vi "Combine_Anomaly_Detection_Results.vi"(4 "Relative Resolution":sgl=1.0, 5 "Evaluation_Results":T7={"Threshold(Image)"=-1.0, "Threshold(Pixel)"=-1.0, "Pixel_Range"={"Min"=-1.0, "Max"=-1.0}} {"Pixel_Range"."Min" format="%#_5g"}, 6 "Display_Options":T1={"ROI_Options"={"Color"=16711680, "Width"=3, "Drawing Mode"=enum."Frame"}, "Heatmap_Options"={"ColorMap"=enum."Jet", "Alpha"=0.4, "Heatmap Range"={"Min"=-1.0, "Max"=-1.0}}, "Has GT?"=FALSE} {"Heatmap_Options"."Heatmap Range"."Min" format="%#_5g"}, 7 "Pixel Anomaly Thrshld":sgl=26.0 format="%_4g", 8 "error in":errorcluster, 9 "Anomaly Map":sgl[][](array[numeric]), 10 "Gt File Path":path, 11 "Orig Image In":T6=refnum) -> (0 "error out":errorcluster, 2 "Actual Pixel Threshold":sgl=26.0, 3 "Anomaly Detection Rresults":T8={"Image"="remote image 000002ADCD8F5788", "Ground Truth"=refnum, "Predicted Heat Map"="remote image 000002ADCD8F5838", "Predicted Mask"="remote image 000002ADCD8F5A48", "Segmentation"=refnum})   [LabVIEW 2020]
uses:
  Controls/Anomaly_Detection_Results_Imgs.ctl
  <vilib>/Ngene/DeepLTK Anomaly Detection Addon/DeepLTK_Anomaly_Detection_Addon/API/Controls/NNPC_Evaluation_Results.ctl
  <vilib>/vision/Image Controls.llb/IMAQ Image.ctl
  Controls/Display_Options.ctl
  Controls/ROI_Display_Options.ctl
  Controls/Heatmap_Display_Options.ctl
  Controls/ColorMap.ctl
  <vilib>/Ngene/DeepLTK Anomaly Detection Addon/DeepLTK_Anomaly_Detection_Addon/API/Controls/MinMax.ctl
  <vilib>/vision/NI_Vision_Development_Module.lvlib
  <vilib>/Ngene/DeepLTK Anomaly Detection Addon/DeepLTK_Anomaly_Detection_Addon/DeepLTK_Anomaly_Detection_Addon.lvlib
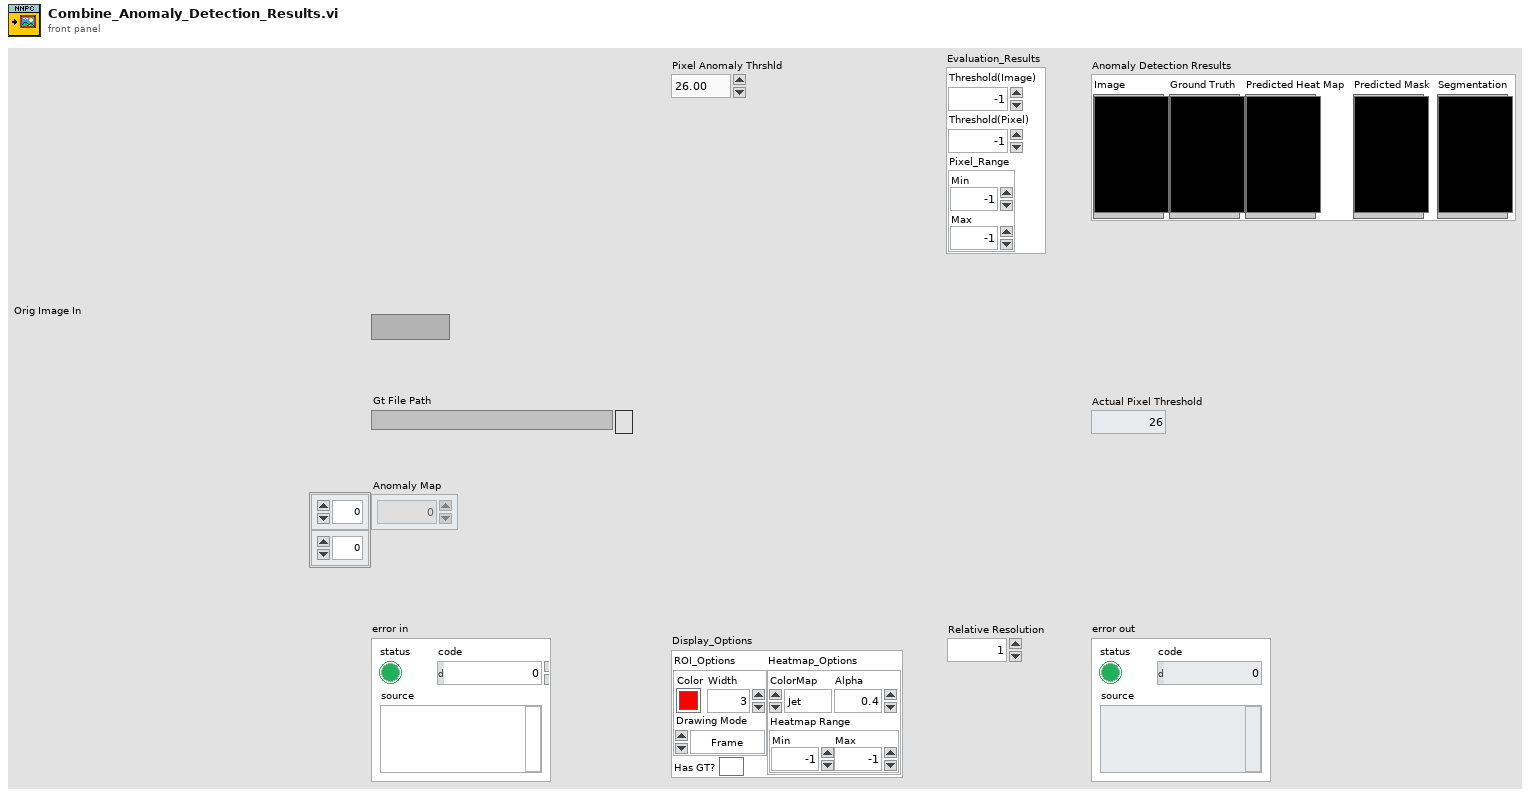
[diagram p1: front panel]
types:
  T1 = typedef "Display_Options.ctl" = cluster{"ROI_Options":T2, "Heatmap_Options":T3, "Has GT?":bool}
  T2 = typedef "ROI_Display_Options.ctl" = cluster{"Color":u32, "Width":u32, "Drawing Mode":enum16{"Frame", "Fill"}}
  T3 = typedef "Heatmap_Display_Options.ctl" = cluster{"ColorMap":T4, "Alpha":sgl, "Heatmap Range":T5}
  T4 = typedef "ColorMap.ctl" = enum16{"Jet", "Perula", "Inferno", "Plasma", "Viridis"}
  T5 = typedef "DeepLTK_Anomaly_Detection_Addon.lvlib/MinMax.ctl" = cluster{"Min":sgl, "Max":sgl}
  T6 = typedef "IMAQ Image.ctl" = refnum<image>
  T7 = typedef "DeepLTK_Anomaly_Detection_Addon.lvlib/NNPC_Evaluation_Results.ctl" = cluster{"Threshold(Image)":sgl, "Threshold(Pixel)":sgl, "Pixel_Range":cluster{"Min":sgl, "Max":sgl}}
  T8 = typedef "Anomaly_Detection_Results_Imgs.ctl" = cluster{"Image":T6, "Ground Truth":T6, "Predicted Heat Map":T6, "Predicted Mask":T6, "Segmentation":T6}
  T9 = typedef "Image Type" = u32
  T10 = typedef "ROI Descriptor" = cluster{"Global Rectangle":i32[], "Contours":cluster{"ID":enum32{"External", "Internal"}, "Type":u32, "Coordinates":i32[]}[]}
  T11 = cluster{"ID":enum32{"External", "Internal"}, "Type":u32, "Coordinates":i32[]}[]
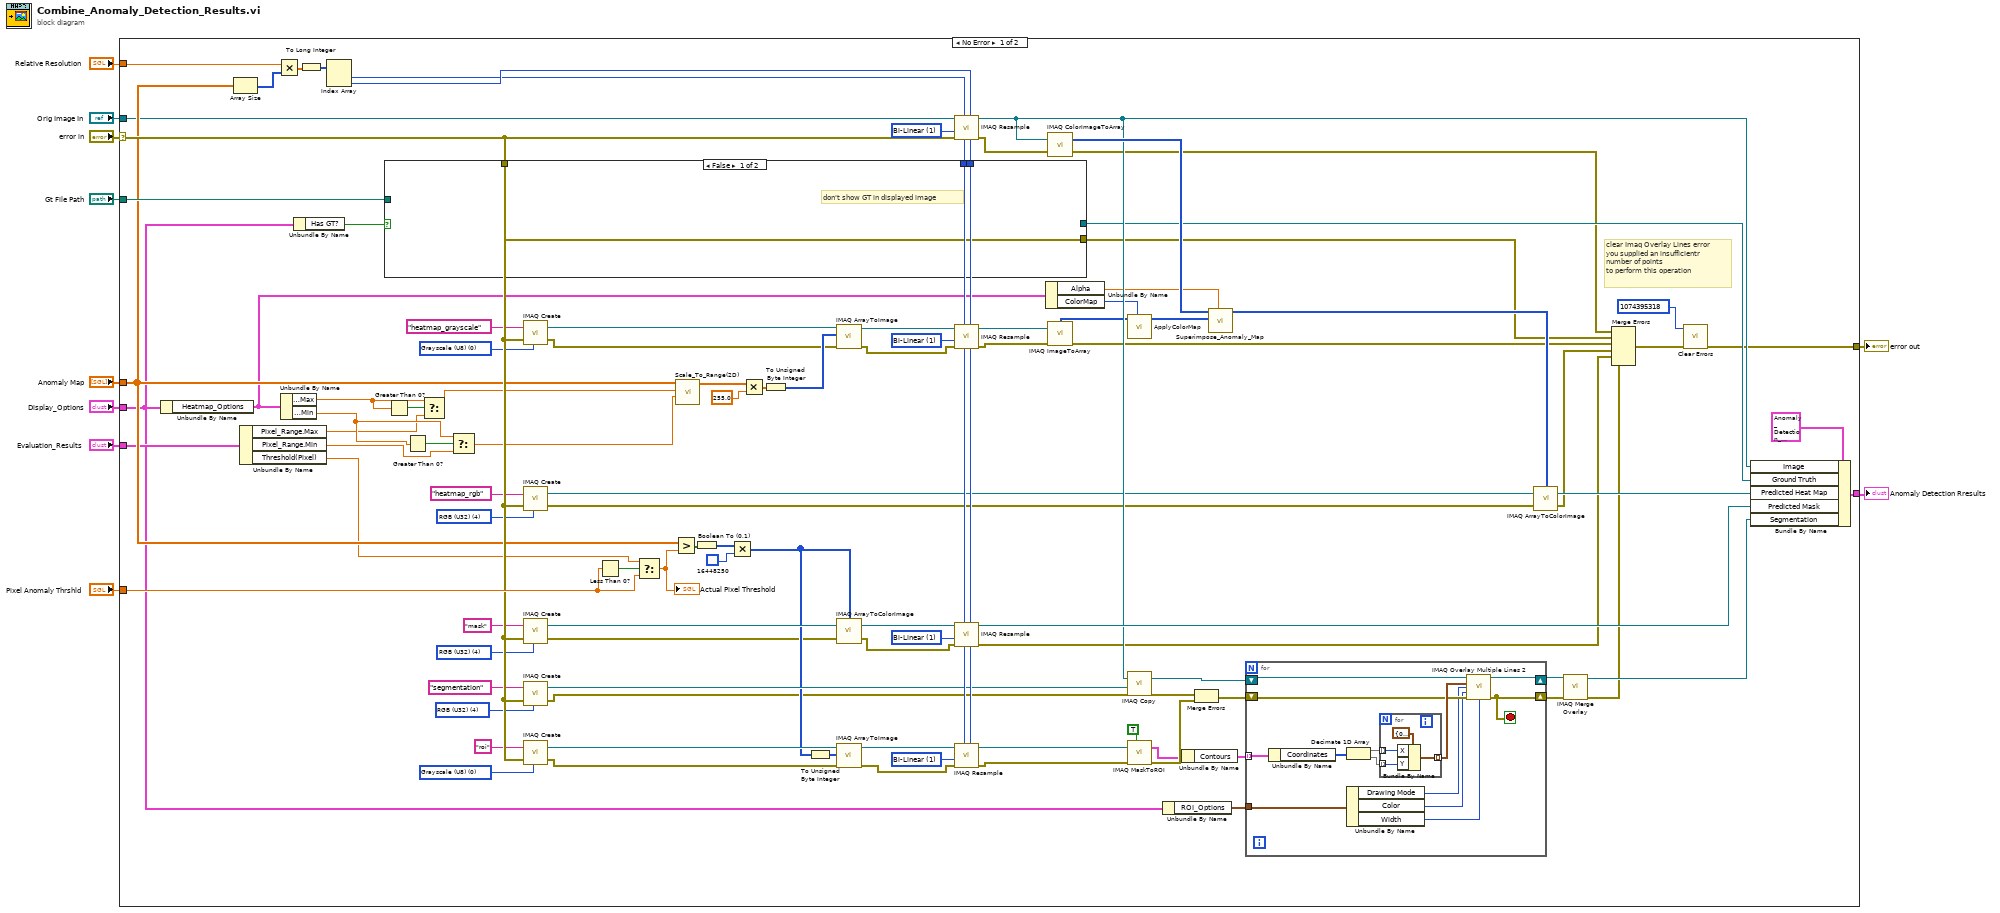
[diagram p0: block diagram]
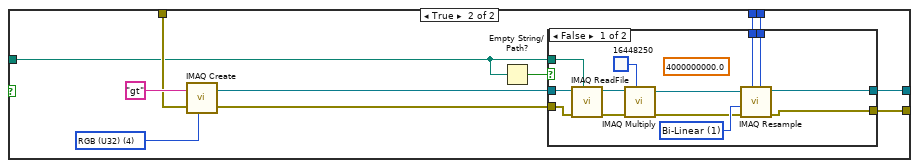
[diagram p2: hidden frame]
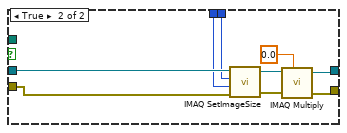
[diagram p3: hidden frame]
diagram:
  n1 = case shown="No Error" "error in" {
    selector: "error in" -> [w101 w164]
    tunnel: [w110 _] -> w10
    tunnel: "Display_Options" -> [w15 _]
    tunnel: "Pixel Anomaly Thrshld" -> [w106 _]
    tunnel: "Gt File Path" -> [w100 _]
    tunnel: [w11 w164] -> w6
    tunnel: "Anomaly Map" -> [w99 _]
    tunnel: "Evaluation_Results" -> [w98 _]
    tunnel: "Relative Resolution" -> [w97 _]
    tunnel: "Orig Image In" -> [w91 _]
    frame No Error {
      w51 = u32 1 items=["Zero Order", "Bi-Linear", "Quadratic", "Cubic Spline"] ("Interpolation Type")
      w59 = u32 1 items=["Zero Order", "Bi-Linear", "Quadratic", "Cubic Spline"] ("Interpolation Type")
      w63 = T9 0 items=["Grayscale (U8)", "Grayscale (I16)", "Grayscale (SGL)", "Complex (CSG)", "RGB (U32)", "HSL (U32)", "RGB (U64)", "Grayscale (U16)"] ("Image Type")
      w70 = u32 1 items=["Zero Order", "Bi-Linear", "Quadratic", "Cubic Spline"] ("Interpolation Type")
      w75 = T9 4 items=["Grayscale (U8)", "Grayscale (I16)", "Grayscale (SGL)", "Complex (CSG)", "RGB (U32)", "HSL (U32)", "RGB (U64)", "Grayscale (U16)"] ("Image Type")
      w78 = T9 4 items=["Grayscale (U8)", "Grayscale (I16)", "Grayscale (SGL)", "Complex (CSG)", "RGB (U32)", "HSL (U32)", "RGB (U64)", "Grayscale (U16)"] ("Image Type")
      w80 = T9 4 items=["Grayscale (U8)", "Grayscale (I16)", "Grayscale (SGL)", "Complex (CSG)", "RGB (U32)", "HSL (U32)", "RGB (U64)", "Grayscale (U16)"] ("Image Type")
      w89 = T9 0 items=["Grayscale (U8)", "Grayscale (I16)", "Grayscale (SGL)", "Complex (CSG)", "RGB (U32)", "HSL (U32)", "RGB (U64)", "Grayscale (U16)"] ("Image Type")
      w103 = u32 1 items=["Zero Order", "Bi-Linear", "Quadratic", "Cubic Spline"] ("Interpolation Type")
      # "clear Imaq Overlay Lines error\nyou supplied an insufficientr number of points\nto perform this operation"
      n2 = Unbundle By Name(w15) -> ("Heatmap_Options"=w17:T3)
      n3 = Array Size(array=w99) -> (size(s)=w92:i32[])
      n4 = Unbundle By Name(w98) -> ("Pixel_Range.Max"=w32:sgl, "Pixel_Range.Min"=w31:sgl, "Threshold(Pixel)"=w30:sgl)
      n5 = Multiply(x=w97, y=w92) -> (x*y=w94:sgl[])
      n6 = Unbundle By Name(w17) -> ("Heatmap Range.Max"=w33:sgl, "Heatmap Range.Min"=w34:sgl)
      n7 = Unbundle By Name(w15) -> ("Has GT?"=w16:bool)
      n8 = To Long Integer(number=w94) -> (32bit integer=w93:i32[])
      n9 = Index Array(array=w93) -> (element #1=w95:i32, element #2=w96:i32)  [unwired: 2 in]
      n10 = case shown="False" w16 {
        tunnel: [_ w122] -> w104
        tunnel: w101 -> [w113 w119]
        tunnel: w100 -> [_ w118]
        tunnel: w96 -> [_ w116]
        tunnel: w95 -> [_ w115]
        tunnel: [w113 w114] -> w19
        frame False {
          # "don't show GT in displayed image"
        }
        frame True {
          w123 = T9 4 items=["Grayscale (U8)", "Grayscale (I16)", "Grayscale (SGL)", "Complex (CSG)", "RGB (U32)", "HSL (U32)", "RGB (U64)", "Grayscale (U16)"] ("Image Type")
          n11 = call "IMAQ Create"("Image Name"="gt", "Image Type"=w123, "error in (no error)"=w119) -> ("New Image"=w120:T6, "error out"=w117:errorcluster)  [unwired: 2 in]
          n12 = Empty String/Path?(string/path=w118) -> (empty?=w121:bool)
          n13 = case shown="False" w121 {
            tunnel: w120 -> [w137 w146]
            tunnel: w118 -> [w136 _]
            tunnel: [w135 w140] -> w122
            tunnel: [w134 w139] -> w114
            tunnel: w116 -> [w133 w145]
            tunnel: w115 -> [w132 w144]
            tunnel: w117 -> [w130 w138]
            frame False {
              (unwired) 4000000000.0 ("Constant")
              w131 = u32 1 items=["Zero Order", "Bi-Linear", "Quadratic", "Cubic Spline"] ("Interpolation Type")
              n14 = call "IMAQ ReadFile"("File Path"=w136, "error in (no error)"=w130, "Image"=w137) -> ("error out"=w128:errorcluster, "Image Out"=w129:T6)  [unwired: 4 in, 3 out]
              n15 = call "IMAQ Multiply"("Image Src A"=w129, "Constant"=u32 16448250, "error in (no error)"=w128) -> ("Image Dst Out"=w126:T6, "error out"=w127:errorcluster)  [unwired: 4 in]
              n16 = call "IMAQ Resample"("X Resolution"=w133, "Y Resolution"=w132, "error in (no error)"=w127, "Interpolation Type"=w131, "Image Src"=w126) -> ("error out"=w134:errorcluster, "Image Dst Out"=w135:T6)  [unwired: 5 in]
            }
            frame True {
              n17 = call "IMAQ SetImageSize"("error in (no error)"=w138, "Y Resolution"=w144, "X Resolution"=w145, "Image"=w146) -> ("error out"=w143:errorcluster, "Image Out"=w142:T6)  [unwired: 1 in]
              n18 = call "IMAQ Multiply"("Image Src A"=w142, "Constant"=0.0, "error in (no error)"=w143) -> ("Image Dst Out"=w140:T6, "error out"=w139:errorcluster)  [unwired: 4 in]
            }
          }
        }
      }
      n19 = Greater Than 0?(x=w33) -> (x > 0?=w37:bool)
      n20 = Greater Than 0?(x=w34) -> (x > 0?=w35:bool)
      n21 = Select(t=w33, s=w37, f=w32) -> (s? t:f=w38:sgl)
      n22 = Select(t=w34, s=w35, f=w31) -> (s? t:f=w36:sgl)
      n23 = call "IMAQ Create"("Image Name"="heatmap_grayscale", "Image Type"=w63, "error in (no error)"=w101) -> ("New Image"=w62:T6, "error out"=w47:errorcluster)  [unwired: 2 in]
      n24 = call "IMAQ Create"("Image Name"="heatmap_rgb", "Image Type"=w80, "error in (no error)"=w101) -> ("New Image"=w79:T6, "error out"=w42:errorcluster)  [unwired: 2 in]
      n25 = call "IMAQ Create"("Image Name"="mask", "Image Type"=w78, "error in (no error)"=w101) -> ("New Image"=w76:T6, "error out"=w49:errorcluster)  [unwired: 2 in]
      n26 = call "IMAQ Create"("Image Name"="segmentation", "Image Type"=w75, "error in (no error)"=w101) -> ("New Image"=w73:T6, "error out"=w43:errorcluster)  [unwired: 2 in]
      n27 = call "IMAQ Create"("Image Name"="roi", "Image Type"=w89, "error in (no error)"=w101) -> ("New Image"=w88:T6, "error out"=w44:errorcluster)  [unwired: 2 in]
      n28 = Less Than 0?(x=w106) -> (x < 0?=w53:bool)
      n29 = Select(t=w30, s=w53, f=w106) -> (s? t:f=w50:sgl)
      "Actual Pixel Threshold" <- w50
      n30 = Greater?(x=w99, y=w50) -> (0:w84:bool[][])
      n31 = call "Scale_To_Range(2D).vi"("min pixel score"=w36, "max pixel score"=w38, "anomaly map"=w99) -> ("anomaly map normalized"=w87:sgl[][])  [unwired: 8 in]
      n32 = Boolean To (0,1)(Boolean=w84) -> (0, 1=w85:i16[][])
      n33 = Multiply(x=w85, y=u32 16448250) -> (x*y=w72:u32[][])
      n34 = Multiply(x=w87, y=sgl 255.0) -> (x*y=w66:sgl[][])
      n35 = To Unsigned Byte Integer(number=w66) -> (unsigned 8bit integer=w65:u8[][])
      n36 = To Unsigned Byte Integer(number=w72) -> (unsigned 8bit integer=w67:u8[][])
      n37 = call "IMAQ ArrayToImage"("error in (no error)"=w47, "Image Pixels (U8)"=w65, "Image"=w62) -> ("error out"=w48:errorcluster, "Image Out"=w61:T6)  [unwired: 7 in]
      n38 = call "IMAQ ArrayToColorImage"("Image Pixels (U32)"=w72, "Image"=w76, "error in (no error)"=w49) -> ("Image Out"=w69:T6, "error out"=w46:errorcluster)  [unwired: 2 in]
      n39 = call "IMAQ ArrayToImage"("error in (no error)"=w44, "Image Pixels (U8)"=w67, "Image"=w88) -> ("error out"=w45:errorcluster, "Image Out"=w55:T6)  [unwired: 7 in]
      n40 = call "IMAQ Resample"("X Resolution"=w96, "Y Resolution"=w95, "error in (no error)"=w101, "Interpolation Type"=w103, "Image Src"=w91) -> ("error out"=w102:errorcluster, "Image Dst Out"=w105:T6)  [unwired: 5 in]
      n41 = call "IMAQ Resample"("X Resolution"=w96, "Y Resolution"=w95, "error in (no error)"=w48, "Interpolation Type"=w59, "Image Src"=w61) -> ("error out"=w58:errorcluster, "Image Dst Out"=w60:T6)  [unwired: 5 in]
      n42 = call "IMAQ Resample"("X Resolution"=w96, "Y Resolution"=w95, "error in (no error)"=w46, "Interpolation Type"=w70, "Image Src"=w69) -> ("error out"=w41:errorcluster, "Image Dst Out"=w107:T6)  [unwired: 5 in]
      n43 = call "IMAQ Resample"("X Resolution"=w96, "Y Resolution"=w95, "error in (no error)"=w45, "Interpolation Type"=w51, "Image Src"=w55) -> ("error out"=w54:errorcluster, "Image Dst Out"=w56:T6)  [unwired: 5 in]
      n44 = Unbundle By Name(w17) -> ("Alpha"=w21:sgl, "ColorMap"=w20:T4)
      n45 = call "IMAQ ColorImageToArray"("Image"=w105, "error in (no error)"=w102) -> ("Image Pixels (U32)"=w111:u32[][], "error out"=w18:errorcluster)  [unwired: 2 in, 1 out]
      n46 = call "IMAQ ImageToArray"("error in (no error)"=w58, "Image"=w60) -> ("error out"=w39:errorcluster, "Image Pixels (U8)"=w57:u8[][])  [unwired: 2 in, 3 out]
      n47 = call "ApplyColorMap.vi"("ColorMap Type"=w20, "Image in"=w57) -> ("Image out"=w71:u32[][])  [unwired: 9 in]
      n48 = call "IMAQ Copy"("error in (no error)"=w43, "Image Dst"=w73, "Image Src"=w105) -> ("error out"=w29:errorcluster, "Image Dst Out"=w26:T6)  [unwired: 3 in]
      n49 = call "IMAQ MaskToROI"("External edges only (T)"=TRUE, "Image"=w56, "error in (no error)"=w54) -> ("ROI Descriptor"=w28:T10, "error out"=w52:errorcluster)  [unwired: 4 in, 1 out]
      n50 = Unbundle By Name(w15) -> ("ROI_Options"=w22:T2)
      n51 = Unbundle By Name(w28) -> ("Contours"=w27:T11)
      n52 = Merge Errors(w29, w52) -> (w24:errorcluster)
      n53 = call "Superimpose_Anomaly_Map.vi"("Alpha"=w21, "Anomaly Map"=w71, "Image"=w111) -> ("Img out"=w82:u32[][])  [unwired: 8 in]
      n54 = for {
        tunnel: w27 -> [w159] mode=indexing
        shift-right: [w147] -> w23
        shift-left: w24 -> [w152]
        tunnel: w22 -> [w151]
        shift-right: [w153] -> w25
        shift-left: w26 -> [w154]
        stop <- w147 stop-if-true
        n55 = Unbundle By Name(w159) -> ("Coordinates"=w158:i32[])
        n56 = Decimate 1D Array(w158) -> (w157:i32[], w156:i32[])
        n57 = Unbundle By Name(w151) -> ("Drawing Mode"=w150:enum16{"Frame", "Fill"}, "Color"=w149:u32, "Width"=w148:u32)
        n58 = for {
          tunnel: w157 -> [w162] mode=indexing
          tunnel: w156 -> [w161] mode=indexing
          tunnel: [w160] -> w155 mode=indexing
          n59 = Bundle By Name(cluster=cluster{"X":dbl, "Y":dbl} {"X"=0.0, "Y"=0.0} ("Line End Points"), "X"=w162, "Y"=w161) -> (w160:cluster{"X":dbl, "Y":dbl})
        }
        n60 = call "IMAQ Overlay Multiple Lines 2"("Image"=w154, "Line End Points"=w155, "Drawing Mode (Frame)"=w150, "Color"=w149, "error in (no error)"=w152, "Width"=w148) -> ("Image Out"=w153:T6, "error out"=w147:errorcluster)  [unwired: 8 in]
      }
      n61 = call "IMAQ ArrayToColorImage"("Image Pixels (U32)"=w82, "Image"=w79, "error in (no error)"=w42) -> ("Image Out"=w108:T6, "error out"=w40:errorcluster)  [unwired: 2 in]
      n62 = call "IMAQ Merge Overlay"("error in (no error)"=w23, "Image Src"=w25) -> ("error out"=w13:errorcluster, "Image Dst Out"=w109:T6)  [unwired: 8 in]
      n63 = Merge Errors(w18, w19, w39, w40, w41, w13) -> (w12:errorcluster)
      n64 = call <vilib>:"Clear Errors.vi"("error in (no error)"=w12, "specific error code to clear (0: all)"=1074395318) -> ("error out"=w11:errorcluster)  [unwired: 4 in, 1 out]
      n65 = Bundle By Name(cluster=T8 {"Image"=refnum, "Ground Truth"=refnum, "Predicted Heat Map"=refnum, "Predicted Mask"=refnum, "Segmentation"=refnum} ("Anomaly Detection Results"), "Image"=w105, "Ground Truth"=w104, "Predicted Heat Map"=w108, "Predicted Mask"=w107, "Segmentation"=w109) -> (w110:T8)
    }
    frame Error {
    }
  }
  "error out" <- w6
  "Anomaly Detection Rresults" <- w10
